vi "Select Sensor.vi"(0 "Channel":string, 5 "Sensor Name in":string, 11 "Sensors":T1(array[cluster])) -> (6 "Sensor Name out":string)   [LabVIEW 2023]
panel:
  in  "Cancel Button":bool
  in  "OK Button":bool
  in  "Available Sensors":i32(listbox)
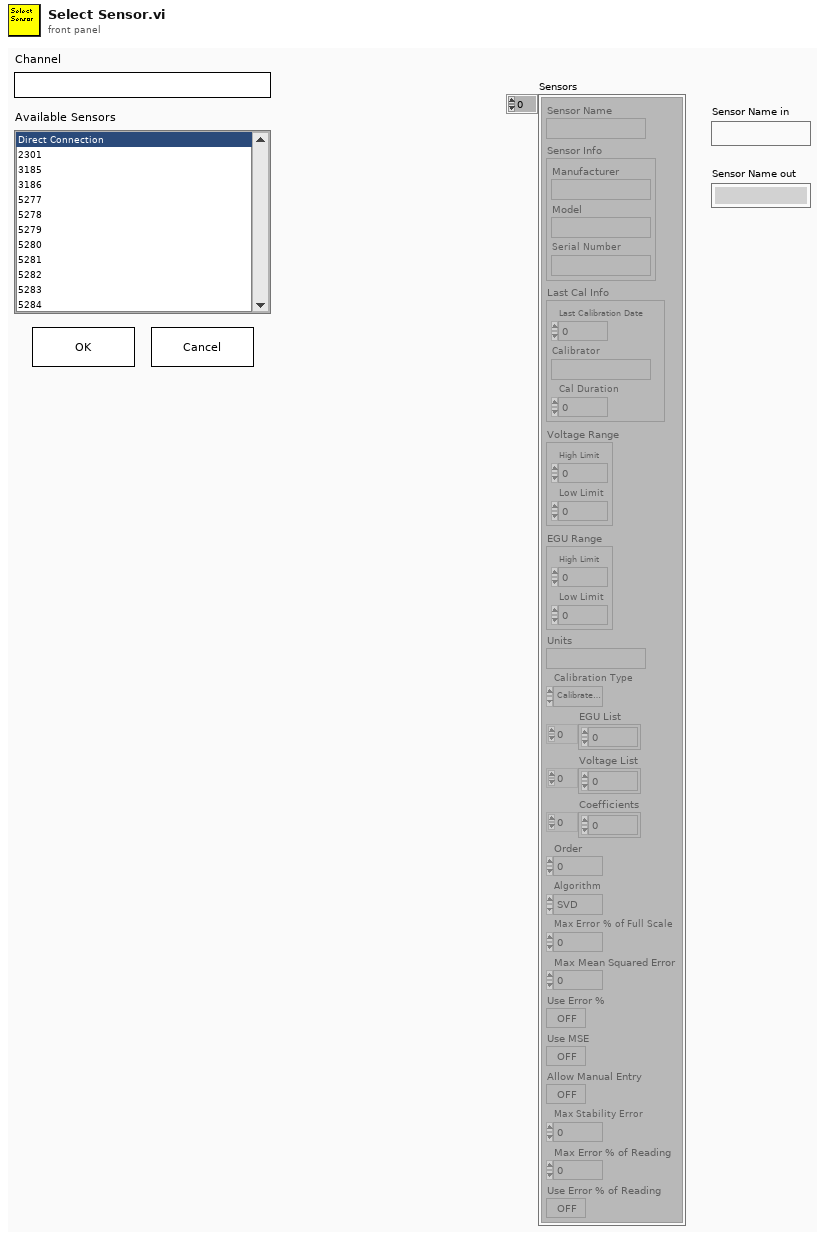
[diagram p1: front panel]
types:
  T1 = cluster{"Sensor Name":string, "Sensor Info":cluster{"Manufacturer":string, "Model":string, "Serial Number":string}, "Last Cal Info":cluster{"Last Calibration Date":dbl, "Calibrator":string, "Cal Duration":i32}, "Voltage Range":cluster{"High Limit":dbl, "Low Limit":dbl}, "EGU Range":cluster{"High Limit":dbl, "Low Limit":dbl}, "Units":string, "Calibration Type":enum16{"Calibrate Analog", "Compare Analog Calibration"}, "EGU List":dbl[], "Voltage List":dbl[], "Coefficients":dbl[], "Order":i32, "Algorithm":enum32{"SVD", "Givens", "Givens2", "Householder", "LU Decomposition", "Cholesky"}, "Max Error % of Full Scale":dbl, "Max Mean Squared Error":dbl, "Use Error %":bool, "Use MSE":bool, "Allow Manual Entry":bool, "Max Stability Error":dbl, "Max Error % of Reading":dbl, "Use Error % of Reading":bool}[]
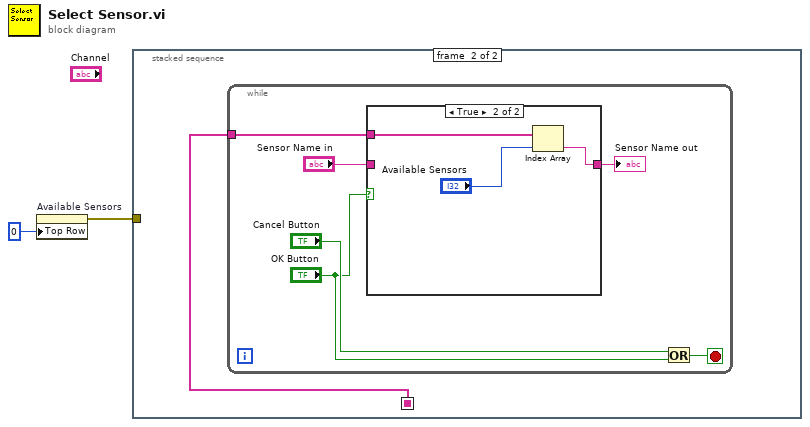
[diagram p0: block diagram]
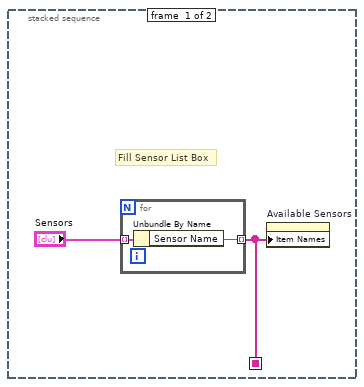
[diagram p2: hidden frame]
diagram:
  n1 = property on="Available Sensors" class="LstBox (strict)"("Top Row"=0 ("Active Row:Active Row Number")) -> (error out=w1:errorcluster)  [unwired: 2 in, 1 out]
  n2 = stacked-sequence {
    seq-local: [w3 _] -> [_ w7]
    tunnel: w1 -> [_ _]
    frame #0 {
      # "Fill Sensor List Box"
      n3 = for {
        tunnel: "Sensors" -> [w6] mode=indexing
        tunnel: [w5] -> w3 mode=indexing
        n4 = Unbundle By Name(w6) -> ("Sensor Name"=w5:string)
      }
      n5 = property on="Available Sensors" class="LstBox (strict)"("Item Names"=w3) -> ()  [unwired: 2 in, 2 out]
    }
    frame #1 {
      n6 = while {
        tunnel: w7 -> [w8]
        stop <- w13 stop-if-true
        n7 = case shown="True" "OK Button" {
          tunnel: "Sensor Name in" -> [w14 _]
          tunnel: [w14 w16] -> w9
          tunnel: w8 -> [_ w17]
          frame False {
          }
          frame True {
            n8 = Index Array(array=w17, index="Available Sensors") -> (element=w16:string)
          }
        }
        "Sensor Name out" <- w9
        n9 = Or(x="Cancel Button", y="OK Button") -> (x .or. y?=w13:bool)
      }
    }
  }
